vi "제목없음 1.vi"() -> ()   [LabVIEW 2014]
uses:
  <vilib>/Utility/sysdir.llb/System Directory Type.ctl
panel:
  out "경로":path
  out "원소":i32
  out "활주로":string[](array[string])
  in  "문자열":string="RKSI"
  out "x-y":i32
  out "바람계산":i32[](array[numeric])
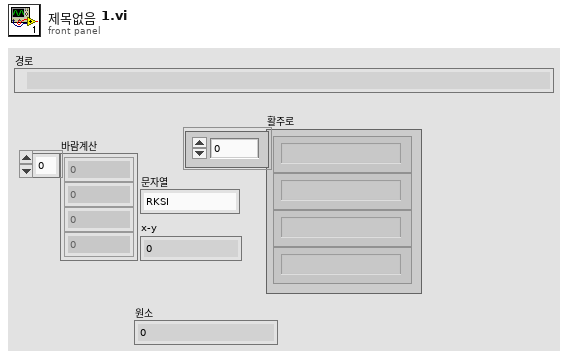
[diagram p1: front panel]
types:
  T1 = enum16{"open", "replace", "create", "open or create", "replace or create", "replace or create with confirmation"}
  T2 = typedef "System Directory Type.ctl" = i32
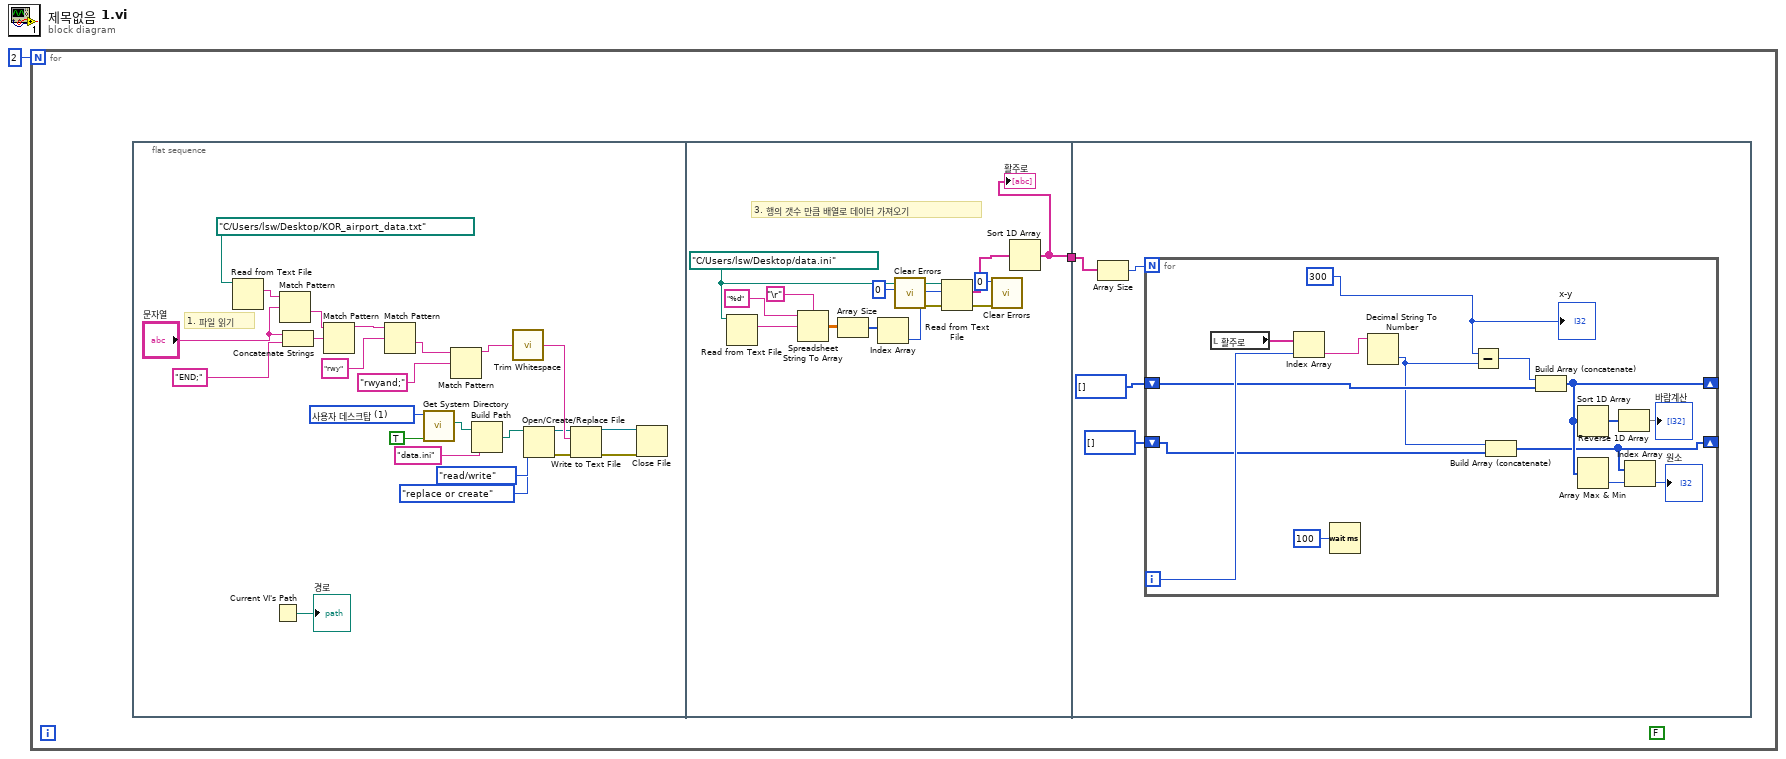
[diagram p0: block diagram]
diagram:
  n1 = for {
    N: 2 -> [_]
    (unwired) FALSE
    n2 = flat-sequence {
      tunnel: [w27] -> w2
      tunnel: w2 -> [w41]
      frame #0 {
        w10 = T2 1 items=["사용자 홈"=0, "사용자 데스크탑"=1, "사용자 문서"=2, "사용자 어플리케이션 데이터"=3, "사용자 환경"=4, "사용자 임시"=5, "퍼블릭 문서"=6, "퍼블릭 어플리케이션 데이터"=7, "퍼블릭 환경"=8, "퍼블릭 캐시"=13, "시스템 코어 라이브러리"=9, "시스템 설치된 라이브러리"=10, "어플리케이션 파일"=11, "부팅 볼륨 루트"=12] ("system directory type")
        # "1. 파일 읽기"
        n3 = Read from Text File(file (use dialog)=path "C:/Users/lsw/Desktop/KOR_airport_data.txt" ("File Path Control")) -> (text=w23:string)  [unwired: 1 in, 5 out]
        n4 = Current VI's Path() -> (path=→"경로":path)
        n5 = Match Pattern(string=w23, regular expression="문자열") -> (after substring=w24:string)  [unwired: 1 in, 3 out]
        n6 = Concatenate Strings("문자열", "END;" ("정규식")) -> (w21:string)
        n7 = Match Pattern(string=w24, regular expression=w21) -> (before substring=w22:string)  [unwired: 1 in, 3 out]
        n8 = Match Pattern(string=w22, regular expression="rwy" ("문자열")) -> (after substring=w18:string)  [unwired: 1 in, 3 out]
        n9 = call <vilib>:"Get System Directory.vi"("create directory if not found? (F)"=TRUE, "system directory type"=w10) -> ("system directory"=w11:path)  [unwired: 9 in]
        n10 = Match Pattern(string=w18, regular expression="rwyand;" ("정규식")) -> (before substring=w16:string)  [unwired: 1 in, 3 out]
        n11 = Build Path(base path=w11, name or relative path="data.ini" ("이름 또는 상대 경로")) -> (appended path=w12:path)
        n12 = call <vilib>:"Trim Whitespace.vi"("string"=w16) -> ("trimmed string"=w15:string)  [unwired: 1 in]
        n13 = Open/Create/Replace File(file path (use dialog)=w12, operation (0:open)=T1."replace or create" ("동작(0:open)"), access (0:read/write)=enum16{"read/write", "read-only", "write-only"}."read/write" ("접근(0:읽기/쓰기)")) -> (refnum out=w7:refnum<file>, error out=w14:errorcluster)  [unwired: 3 in, 1 out]
        n14 = Write to Text File(file (use dialog)=w7, text=w15, error in=w14) -> (refnum out=w8:refnum<file>, error out=w13:errorcluster)  [unwired: 1 in, 1 out]
        n15 = Close File(refnum=w8, error in=w13) -> ()  [unwired: 2 out]
      }
      frame #1 {
        w38 = path "C:/Users/lsw/Desktop/data.ini" ("File Path Control")
        # "3. 행의 갯수 만큼 배열로 데이터 가져오기"
        n16 = Read from Text File(file (use dialog)=w38) -> (text=w37:string)  [unwired: 1 in, 5 out]
        n17 = Spreadsheet String To Array(delimiter (Tab)="\r", format string="%d", spreadsheet string=w37) -> (array=w35:dbl[][])  [unwired: 1 out]
        n18 = Array Size(array=w35) -> (size(s)=w36:i32[])
        n19 = Index Array(array=w36) -> (element=w39:i32)  [unwired: 1 in]
        n20 = call <vilib>:"Clear Errors.vi"("specific error code to clear (0: all)"=0) -> ("error out"=w32:errorcluster)  [unwired: 5 in, 1 out]
        n21 = Read from Text File(file (use dialog)=w38, count=w39, error in=w32) -> (text=w28:string[], error out=w30:errorcluster)  [unwired: 3 out]
        n22 = call <vilib>:"Clear Errors.vi"("error in (no error)"=w30, "specific error code to clear (0: all)"=0) -> ()  [unwired: 4 in, 2 out]
        n23 = Sort 1D Array(array=w28) -> (sorted array=w27:string[])
        "활주로" <- w27
      }
      frame #2 {
        n24 = Array Size(array=w41) -> (size(s)=w42:i32)
        n25 = for {
          N: w42 -> [_]
          shift-right: [w49] -> _
          shift-left: i32[] [] -> [w55]
          shift-right: [w45] -> _
          shift-left: i32[] [] -> [w47]
          i -> [w58]
          w52 = 300
          n26 = local read "활주로"() -> (w54:string[])
          n27 = Index Array(array=w54, index=w58) -> (element=w53:string)
          n28 = Wait (ms)(milliseconds to wait=u32 100 ("대기 시간(ms)")) -> ()  [unwired: 1 out]
          n29 = Decimal String To Number(string=w53) -> (number=w46:i32)  [unwired: 2 in, 1 out]
          n30 = Subtract(x=w52, y=w46) -> (x-y=w56:i32)
          n31 = Build Array (concatenate)(w46, w47) -> (w45:i32[])
          n32 = Build Array (concatenate)(w56, w55) -> (w49:i32[])
          n33 = Sort 1D Array(array=w49) -> (sorted array=w50:i32[])
          n34 = Array Max & Min(array=w49) -> (min index (indices)=w48:i32)  [unwired: 3 out]
          n35 = Reverse 1D Array(array=w50) -> (reversed array=→"바람계산":i32[])
          n36 = Index Array(array=w45, index=w48) -> (element=→"원소":i32)
          "x-y" <- w52
        }
      }
    }
  }
